vi "cal_visa_in_error_in_pos.vi"(10 "Last Function Position":cluster{"Left":i32, "Top":i32}, 11 "Last Control Position":cluster{"Left":i32, "Top":i32}) -> (2 "Error In Position":cluster{"Left":i32, "Top":i32}, 3 "Visa In Position":cluster{"Left":i32, "Top":i32})   [LabVIEW 2018]
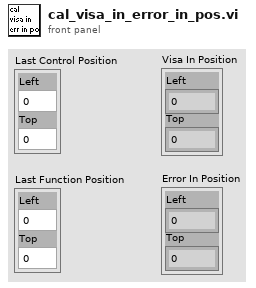
[diagram p1: front panel]
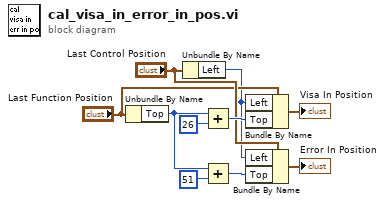
[diagram p0: block diagram]
diagram:
  n1 = Unbundle By Name("Last Function Position") -> ("Top"=w2:i32)
  n2 = Unbundle By Name("Last Control Position") -> ("Left"=w1:i32)
  n3 = Add(x=w2, y=26) -> (x+y=w9:i32)
  n4 = Add(x=w2, y=51) -> (x+y=w3:i32)
  n5 = Bundle By Name(cluster="Last Function Position", "Left"=w1, "Top"=w9) -> (→"Visa In Position":cluster{"Left":i32, "Top":i32})
  n6 = Bundle By Name(cluster="Last Control Position", "Left"=w1, "Top"=w3) -> (→"Error In Position":cluster{"Left":i32, "Top":i32})
